vi "Decode Error.vi"(8 "error in (no error)":errorcluster, 10 "Enable MSS Bit Set (F: Disable)":bool, 11 "VISA resource name":refnum<visa-resource-name>) -> (0 "error out":errorcluster, 2 "Error Message":string, 3 "VISA resource name out":refnum<visa-resource-name>)   [LabVIEW 2016, in "Lake Shore 350.lvlib"]
doc: "Called by the 350 Error Query VI. It's function is to query the 350 Status Byte and decode errors if the Status Byte reports errors are present. \n\nNote that the calling VI checks the Status Byte in the case of a timeout error. If the calling VI indicates the Status Byte is already reporting errors, this VI will not query the Status Byte again, it will go straight to the process of decoding errors.\n\nThe following conditions will be returned as errors in the Error Out cluster:\n<B>Processor Communication Error</B>\n<B>Query Error</B>\n<B>Execution Error</B>\n<B>Command Error</B>\n<B>Calibration Error</B>\n\nThe following conditions will be returned as warnings in the Error Out cluster:\n<B>Sensor Alarming</B>\n<B>Invalid Reading</B>\n<B>Temperature Underrange</B>\n<B>Temperature Overrange</B>\n<B>Sensor Units Zero</B>\n<B>Sensor Units Overrange</B>"
uses:
  Lake Shore 350.lvlib
  Instance           1 20Saved   Decode Error .vi
  Instance           2 20Saved   Decode Error .vi
  Instance           3 20Saved   Decode Error .vi
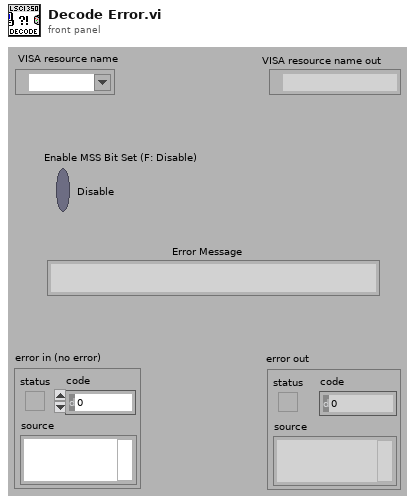
[diagram p1: front panel]
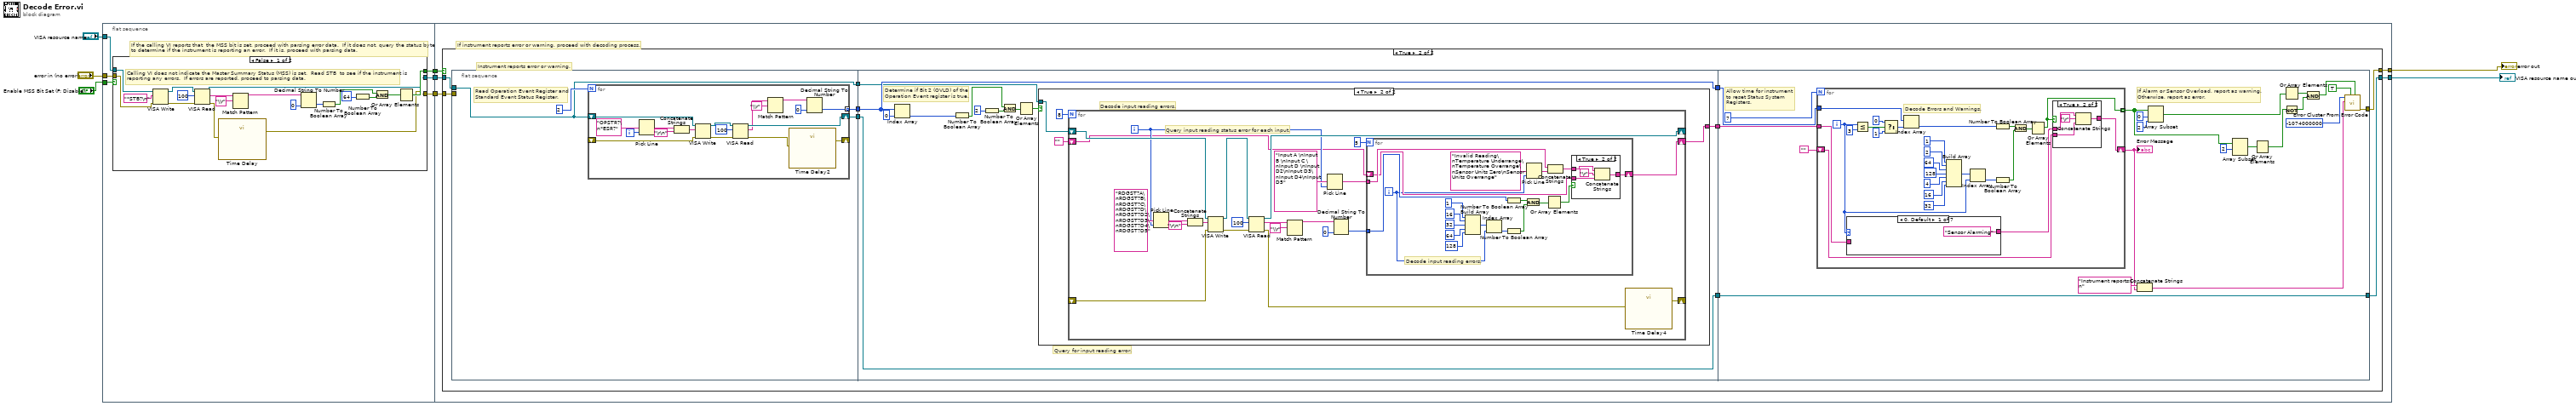
[diagram p0: block diagram]
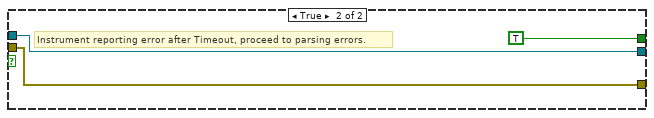
[diagram p2: hidden frame]
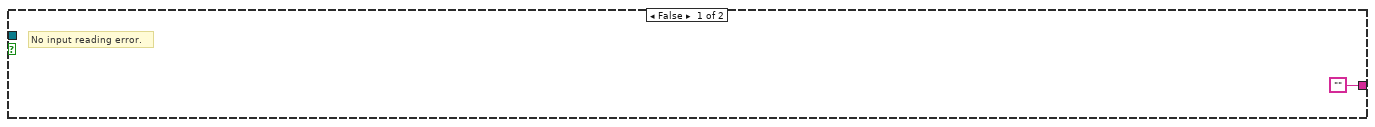
[diagram p4: hidden frame]
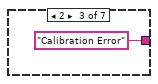
[diagram p7: hidden frame]
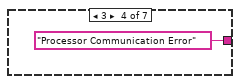
[diagram p8: hidden frame]
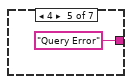
[diagram p9: hidden frame]
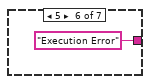
[diagram p10: hidden frame]
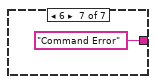
[diagram p11: hidden frame]
diagram:
  n1 = flat-sequence {
    tunnel: "Enable MSS Bit Set (F: Disable)" -> [w14]
    tunnel: "VISA resource name" -> [w13]
    tunnel: "error in (no error)" -> [w12]
    tunnel: [w11] -> w3
    tunnel: [w10] -> w2
    tunnel: [w9] -> w1
    tunnel: [w39] -> w8
    tunnel: [w38] -> w7
    tunnel: w3 -> [w37]
    tunnel: w2 -> [w41]
    tunnel: w1 -> [w40]
    frame #0 {
      # "If the calling VI reports that  the MSS bit is set, proceed with parsing error data.  If it does not, query the status byte\nto determine if the instrument is reporting an error.  If it is, proceed with parsing data."
      n2 = case shown="False" w14 {
        tunnel: w13 -> [w16 w35]
        tunnel: w12 -> [w15 w36]
        tunnel: [w21 TRUE] -> w11
        tunnel: [w17 w36] -> w9
        tunnel: [w20 w35] -> w10
        frame False {
          # "Calling VI does not indicate the Master Summary Status (MSS) is set.  Read STB  to see if the instrument is\nreporting any errors.  If errors are reported, proceed to parsing data."
          n3 = VISA Write(VISA resource name=w16, write buffer="*STB?\n", error in (no error)=w15) -> (VISA resource name out=w31:refnum<visa-resource-name>, error out=w30:errorcluster)  [unwired: 1 out]
          n4 = VISA Read(VISA resource name=w31, byte count=100, error in (no error)=w30) -> (VISA resource name out=w20:refnum<visa-resource-name>, read buffer=w33:string, error out=w18:errorcluster)  [unwired: 1 out]
          n5 = call "Time Delay"("error in (no error)"=w18) -> ("error out"=w17:errorcluster)  [unwired: 10 in]
          n6 = Match Pattern(string=w33, regular expression="\\r") -> (before substring=w26:string)  [unwired: 1 in, 3 out]
          n7 = Decimal String To Number(string=w26, default (0L)=u16 0) -> (number=w19:u16)  [unwired: 1 in, 1 out]
          n8 = Number To Boolean Array(number=w19) -> (Boolean array=w22:bool[])
          n9 = Number To Boolean Array(number=64) -> (Boolean array=w24:bool[])
          n10 = And(x=w22, y=w24) -> (x .and. y?=w23:bool[])
          n11 = Or Array Elements(Boolean array=w23) -> (logical OR=w21:bool)
        }
        frame True {
          # "Instrument reporting error after Timeout, proceed to parsing errors."
        }
      }
    }
    frame #1 {
      # "If instrument reports error or warning, proceed with decoding process."
      n12 = case shown="True" w37 {
        tunnel: w41 -> [w43 w53]
        tunnel: w40 -> [w42 w52]
        tunnel: [w43 w51] -> w39
        tunnel: [w42 w50] -> w38
        frame False {
          # "No instrument error or warning reported."
        }
        frame True {
          # "Instrument reports error or warning."
          n13 = flat-sequence {
            tunnel: w53 -> [w56]
            tunnel: [w56] -> w49
            tunnel: w52 -> [_]
            tunnel: [w55] -> w48
            tunnel: [w54] -> w47
            tunnel: w49 -> [w79]
            tunnel: w48 -> [w76]
            tunnel: [w76] -> w46
            tunnel: w47 -> [w85]
            tunnel: [w85] -> w45
            tunnel: [w78] -> w44
            tunnel: [w139] -> w51
            tunnel: w46 -> [w139]
            tunnel: [w140] -> w50
            tunnel: w45 -> [w143]
            tunnel: w44 -> [w141]
            frame #0 {
              # "Read Operation Event Register and \nStandard Event Status Register."
              n14 = for {
                N: 2 -> [_]
                shift-right: [w73] -> w55
                shift-left: w56 -> [w74]
                shift-right: [w61] -> _
                shift-left: _ -> [w63]
                tunnel: [w64] -> w54 mode=indexing
                i -> [w75]
                n15 = Pick Line(multi-line string="OPSTR?\n*ESR?", line index=w75) -> (output string=w59:string)  [unwired: 1 in]
                n16 = Concatenate Strings(w59, "\r\n") -> (w58:string)
                n17 = VISA Write(VISA resource name=w74, write buffer=w58, error in (no error)=w63) -> (VISA resource name out=w70:refnum<visa-resource-name>, error out=w69:errorcluster)  [unwired: 1 out]
                n18 = VISA Read(VISA resource name=w70, byte count=100, error in (no error)=w69) -> (VISA resource name out=w73:refnum<visa-resource-name>, read buffer=w72:string, error out=w62:errorcluster)  [unwired: 1 out]
                n19 = Match Pattern(string=w72, regular expression="\\r") -> (before substring=w66:string)  [unwired: 1 in, 3 out]
                n20 = call "Time Delay2"("error in (no error)"=w62) -> ("error out"=w61:errorcluster)  [unwired: 10 in]
                n21 = Decimal String To Number(string=w66, default (0L)=u16 0) -> (number=w64:u16)  [unwired: 1 in, 1 out]
              }
            }
            frame #1 {
              # "Query for input reading error."
              # "Determine if Bit 2 (OVLD) of the \nOperation Event register is true."
              n22 = Index Array(array=w85, index=0) -> (element=w86:u16)
              n23 = Number To Boolean Array(number=w86) -> (Boolean array=w81:bool[])
              n24 = Number To Boolean Array(number=2) -> (Boolean array=w80:bool[])
              n25 = And(x=w81, y=w80) -> (x .and. y?=w82:bool[])
              n26 = Or Array Elements(Boolean array=w82) -> (logical OR=w77:bool)
              n27 = case shown="True" w77 {
                tunnel: w79 -> [_ w90]
                tunnel: ["" w88] -> w78
                frame False {
                  # "No input reading error."
                }
                frame True {
                  # "Decode input reading errors."
                  n28 = for {
                    N: 8 -> [_]
                    shift-right: [w113] -> _
                    shift-left: w90 -> [w114]
                    shift-right: [w103] -> _
                    shift-left: _ -> [w105]
                    shift-right: [w92] -> w88
                    shift-left: "" -> [w93]
                    i -> [w97]
                    # "Query input reading status error for each input."
                    n29 = Pick Line(multi-line string="RDGST?A\nRDGST?B\nRDGST?C\nRDGST?D\nRDGST?D2\nRDGST?D3\nRDGST?D4\nRDGST?D5", line index=w97) -> (output string=w101:string)  [unwired: 1 in]
                    n30 = Concatenate Strings(w101, "\r\n") -> (w100:string)
                    n31 = VISA Write(VISA resource name=w114, write buffer=w100, error in (no error)=w105) -> (VISA resource name out=w110:refnum<visa-resource-name>, error out=w109:errorcluster)  [unwired: 1 out]
                    n32 = VISA Read(VISA resource name=w110, byte count=100, error in (no error)=w109) -> (VISA resource name out=w113:refnum<visa-resource-name>, read buffer=w112:string, error out=w104:errorcluster)  [unwired: 1 out]
                    n33 = Match Pattern(string=w112, regular expression="\\r") -> (before substring=w106:string)  [unwired: 1 in, 3 out]
                    n34 = Pick Line(multi-line string="Input A \nInput B \nInput C \nInput D \nInput D2\nInput D3\nInput D4\nInput D5", line index=w97) -> (output string=w94:string)  [unwired: 1 in]
                    n35 = Decimal String To Number(string=w106, default (0L)=u16 0) -> (number=w95:u16)  [unwired: 1 in, 1 out]
                    n36 = for {
                      N: 5 -> [_]
                      tunnel: w95 -> [w127]
                      tunnel: w94 -> [w125]
                      shift-right: [w123] -> w92
                      shift-left: w93 -> [w118]
                      i -> [w117]
                      # "Decode input reading errors."
                      n37 = Build Array(1, 16, 32, 64, 128) -> (w116:i32[])
                      n38 = Index Array(array=w116, index=w117) -> (element=w130:i32)
                      n39 = Number To Boolean Array(number=w127) -> (Boolean array=w131:bool[])
                      n40 = Number To Boolean Array(number=w130) -> (Boolean array=w133:bool[])
                      n41 = And(x=w131, y=w133) -> (x .and. y?=w132:bool[])
                      n42 = Pick Line(multi-line string="Invalid Reading\nTemperature Underrange\nTemperature Overrange\nSensor Units Zero\nSensor Units Overrange", line index=w117) -> (output string=w126:string)  [unwired: 1 in]
                      n43 = Or Array Elements(Boolean array=w132) -> (logical OR=w128:bool)
                      n44 = Concatenate Strings(w125, w126) -> (w124:string)
                      n45 = case shown="True" w128 {
                        tunnel: w118 -> [w134 w135]
                        tunnel: w124 -> [_ w138]
                        tunnel: [w134 w137] -> w123
                        frame False {
                        }
                        frame True {
                          n46 = Concatenate Strings(w138, "\r", w135) -> (w137:string)
                        }
                      }
                    }
                    n47 = call "Time Delay4"("error in (no error)"=w104) -> ("error out"=w103:errorcluster)  [unwired: 10 in]
                  }
                }
              }
            }
            frame #2 {
              # "Allow time for instrument\nto reset Status System\nRegisters."
              # "If Alarm or Sensor Overload, report as warning.\nOtherwise, report as error."
              n48 = for {
                N: 7 -> [_]
                shift-right: [w168] -> w157
                shift-left: "" -> [w169]
                tunnel: w143 -> [w178]
                tunnel: [w170] -> w152 mode=indexing
                tunnel: w141 -> [w161]
                i -> [w163]
                # "Decode Errors and Warnings."
                n49 = case shown="0, Default" w163 {
                  tunnel: ["Sensor Alarming" w186 "Calibration Error" "Processor Communication Error" "Query Error" "Execution Error" "Command Error"] -> w162
                  tunnel: w161 -> [_ w186 _ _ _ _ _]
                  frame 0, Default {
                  }
                  frame 1 {
                  }
                  frame 2 {
                  }
                  frame 3 {
                  }
                  frame 4 {
                  }
                  frame 5 {
                  }
                  frame 6 {
                  }
                }
                n50 = Less Or Equal?(x=w163, y=3) -> (x <= y?=w177:bool)
                n51 = Select(t=0, s=w177, f=1) -> (s? t:f=w174:i32)
                n52 = Index Array(array=w178, index=w174) -> (element=w173:u16)
                n53 = Build Array(1, 2, 64, 128, 4, 16, 32) -> (w181:i32[])
                n54 = Index Array(array=w181, index=w163) -> (element=w180:i32)
                n55 = Number To Boolean Array(number=w173) -> (Boolean array=w182:bool[])
                n56 = Number To Boolean Array(number=w180) -> (Boolean array=w184:bool[])
                n57 = And(x=w182, y=w184) -> (x .and. y?=w183:bool[])
                n58 = Or Array Elements(Boolean array=w183) -> (logical OR=w170:bool)
                n59 = case shown="True" w170 {
                  tunnel: w169 -> [w192 w193]
                  tunnel: w162 -> [_ w196]
                  tunnel: [w192 w195] -> w168
                  frame False {
                  }
                  frame True {
                    n60 = Concatenate Strings(w196, "\r", w193) -> (w195:string)
                  }
                }
              }
              "Error Message" <- w157
              n61 = Concatenate Strings("Instrument reports:\n" ("Source"), w157) -> (w154:string)
              n62 = Array Subset(array=w152, index=0, length=2) -> (w150:bool[])
              n63 = Array Subset(array=w152, index=2) -> (w149:bool[])  [unwired: 1 in]
              n64 = Or Array Elements(Boolean array=w149) -> (logical OR=w147:bool)
              n65 = Or Array Elements(Boolean array=w150) -> (logical OR=w148:bool)
              n66 = Not(x=w147) -> (.not. x?=w146:bool)
              n67 = And(x=w148, y=w146) -> (x .and. y?=w144:bool)
              n68 = call <vilib>:"Error Cluster From Error Code.vi"("is warning? (False)"=w144, "show call chain? (False)"=TRUE, "error message (\"\")"=w154, "error code (0)"=-1074000000 ("Code")) -> ("error out"=w140:errorcluster)  [unwired: 5 in]
            }
          }
        }
      }
    }
  }
  "error out" <- w7
  "VISA resource name out" <- w8
